vi "Stream Update All Sensors.vi"(8 "error in":errorcluster, 11 "UART port in":T9) -> (0 "error out":errorcluster, 1 "sensors":T1={"Bumps + Wheel Drops"={"Wheeldrop Caster"=FALSE, "Wheeldrop Left"=FALSE, "Wheeldrop Right"=FALSE, "Bump Left"=FALSE, "Bump Right"=FALSE}, "Wall"=FALSE, "Cliff Left"=FALSE, "Cliff Front Left"=FALSE, "Cliff Front Right"=FALSE, "Cliff Right"=FALSE, "Wall Signal"=0, "Cliff Left Signal"=0, "Cliff Front Left Signal"=0, "Cliff Front Right Signal"=0, "Cliff Right Signal"=0, "Buttons"={"Advance"=FALSE, "Play"=FALSE}, "Virtual Wall"=FALSE, "# Stream Packets"=0, "Requested Velocity (mm/s)"=0, "Requested Radius (mm)"=0, "Requested Right Wheel Velocity (mm/s)"=0, "Requested Left Wheel Velocity (mm/s)"=0, "Distance (mm)"=0, "Angle (deg)"=0, "Song Playing"=FALSE, "Song Number"=0, "Charging State"=enum."Not Charging", "Voltage (mV)"=0, "Current (mA)"=0, "Battery Temperature (deg C)"=0, "Battery Charge (mAh)"=0, "Battery Capacity (mAh)"=0, "Charging Sources"={"Internal Charger"=FALSE, "Home Base"=FALSE}, "OI Mode"=enum."Off", "Digital Inputs"={"Digital Input 0"=FALSE, "Digital Input 1"=FALSE, "Digital Input 2"=FALSE, "Digital Input 3"=FALSE, "Device Detect"=FALSE}, "Drivers & Wheel Overcurrent"={"Low-Side Driver 0"=FALSE, "Low-Side Driver 1"=FALSE, "Low-Side Driver 2"=FALSE, "Left Wheel"=FALSE, "Right Wheel"=FALSE}, "Analog Signal"=0, "Infrared"=255} {"Infrared" format="%02x"}, 3 "UART port out":T9, 5 "Accumulated Distance (mm)":i32, 7 "Accumulated Angle (deg)":i32)   [LabVIEW 2013]
doc: "Reads data from the UART serial port and updates sensors when packets are available.\n\nThis VI assumes that the robot is streaming all sensor data (sensor group 6).\n\nThis VI accumulates distance and angle whenever a new packet is received. While this simplifies most code, which depends on how far the robot has moved, the developer must take account for rollover of signed 32-bit integers if the application has a long running time.\n\nNote that accumulated distance and angle tend to be extremeley inaccurate, since the iRobot looses fractional components of each when it sends a sensor update, and updates are sent at a high rate, resulting in significant roundoff error.\n\nThis VI reads from, but does not write to, the serial port."
uses:
  Advanced/UART/iRobot UART Port Type.ctl
  Sensor Group 6.ctl
  Bumps + Wheel Drops.ctl
  Buttons.ctl
  Charging State.ctl
  Charging Sources Available.ctl
  OI Mode.ctl
  Cargo Bay Digital Inputs.ctl
  Low-Side Driver + Wheel Overcurrent.ctl
  Advanced/UART/iRobot UART Simple Packet Configuration.ctl
panel:
  # "Electrical: charging, battery, OI mode"
  # "Sensors: bump, cliff, button, wheel drop, wall, virtual wall"
  # "Motion: distance, angle, requested velocity"
  # "Cargo Bay: I/O, overcurrent, infrared"
  # "Song"
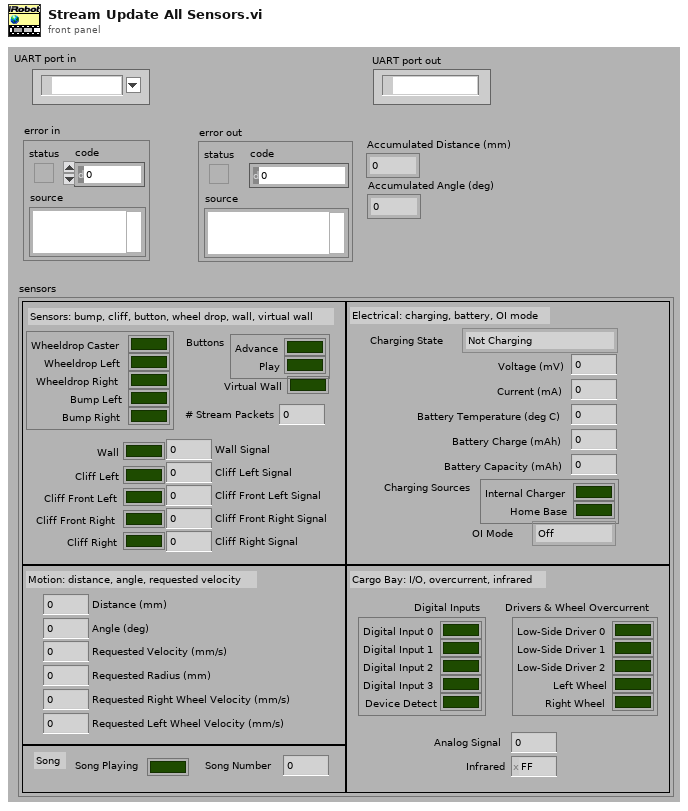
[diagram p1: front panel]
types:
  T1 = typedef "Sensor Group 6.ctl" = cluster{"Bumps + Wheel Drops":T2, "Wall":bool, "Cliff Left":bool, "Cliff Front Left":bool, "Cliff Front Right":bool, "Cliff Right":bool, "Wall Signal":u16, "Cliff Left Signal":u16, "Cliff Front Left Signal":u16, "Cliff Front Right Signal":u16, "Cliff Right Signal":u16, "Buttons":T3, "Virtual Wall":bool, "# Stream Packets":u8, "Requested Velocity (mm/s)":i16, "Requested Radius (mm)":i16, "Requested Right Wheel Velocity (mm/s)":i16, "Requested Left Wheel Velocity (mm/s)":i16, "Distance (mm)":i32, "Angle (deg)":i32, "Song Playing":bool, "Song Number":u8, "Charging State":T4, "Voltage (mV)":u16, "Current (mA)":i16, "Battery Temperature (deg C)":i8, "Battery Charge (mAh)":u16, "Battery Capacity (mAh)":u16, "Charging Sources":T5, "OI Mode":T6, "Digital Inputs":T7, "Drivers & Wheel Overcurrent":T8, "Analog Signal":u16, "Infrared":u8}
  T2 = typedef "Bumps + Wheel Drops.ctl" = cluster{"Wheeldrop Caster":bool, "Wheeldrop Left":bool, "Wheeldrop Right":bool, "Bump Left":bool, "Bump Right":bool}
  T3 = typedef "Buttons.ctl" = cluster{"Advance":bool, "Play":bool}
  T4 = typedef "Charging State.ctl" = enum16{"Not Charging", "Reconditioning Charging", "Full Charging", "Trickle Charging", "Waiting", "Charging Fault Condition"}
  T5 = typedef "Charging Sources Available.ctl" = cluster{"Internal Charger":bool, "Home Base":bool}
  T6 = typedef "OI Mode.ctl" = enum16{"Off", "Passive", "Safe", "Full"}
  T7 = typedef "Cargo Bay Digital Inputs.ctl" = cluster{"Digital Input 0":bool, "Digital Input 1":bool, "Digital Input 2":bool, "Digital Input 3":bool, "Device Detect":bool}
  T8 = typedef "Low-Side Driver + Wheel Overcurrent.ctl" = cluster{"Low-Side Driver 0":bool, "Low-Side Driver 1":bool, "Low-Side Driver 2":bool, "Left Wheel":bool, "Right Wheel":bool}
  T9 = typedef "iRobot UART Port Type.ctl" = refnum<visa-resource-name>
  T10 = typedef "iRobot UART Simple Packet Configuration.ctl" = cluster{"header":u8[], "create checksum?":bool}
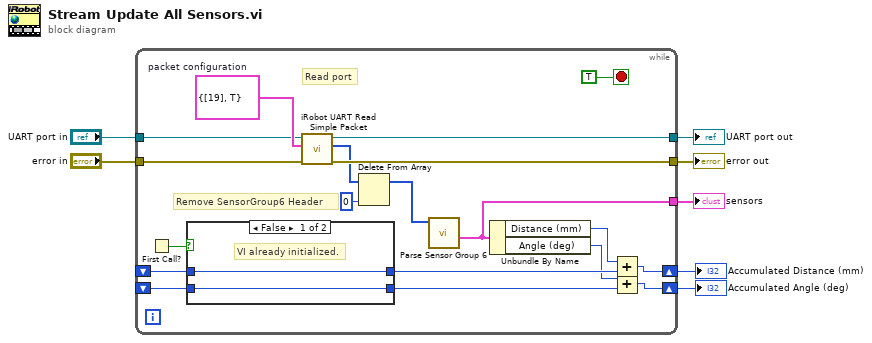
[diagram p0: block diagram]
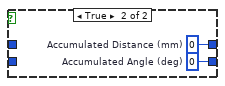
[diagram p2: hidden frame]
diagram:
  n1 = while {
    tunnel: "error in" -> [w13]
    shift-right: [w22] -> w6
    shift-left: _ -> [w20]
    shift-right: [w21] -> w5
    shift-left: _ -> [w19]
    tunnel: [w18] -> w4
    tunnel: [w14] -> w2
    tunnel: "UART port in" -> [w9]
    tunnel: [w8] -> w1
    stop <- TRUE stop-if-true
    w17 = T10 {"header"=[19], "create checksum?"=TRUE}  # packet configuration
    # "Remove SensorGroup6 Header"
    # "Read port"
    n2 = First Call?() -> (First Call?: T/F=w26:bool)
    n3 = case shown="False" w26 {
      tunnel: [w28 w30] -> w24
      tunnel: [w27 w29] -> w23
      tunnel: w20 -> [w28 _]
      tunnel: w19 -> [w27 _]
      frame False {
        # "VI already initialized."
      }
      frame True {
        w29 = 0  # Accumulated Angle (deg)
        w30 = 0  # Accumulated Distance (mm)
      }
    }
    n4 = call "iRobot UART Read Simple Packet.vi"("error in"=w13, "packet configuration"=w17, "UART session"=w9) -> ("error out"=w18:errorcluster, "payload"=w12:u8[], "UART session"=w8:T9)  [unwired: 2 in, 4 out]
    n5 = Delete From Array(array=w12, index=0) -> (array with subset deleted=w10:u8[])  [unwired: 1 in, 1 out]
    n6 = call "Parse Sensor Group 6.vi"("stream in"=w10) -> ("iRobot Sensor Group 6"=w14:T1)  [unwired: 9 in, 1 out]
    n7 = Unbundle By Name(w14) -> ("Distance (mm)"=w16:i32, "Angle (deg)"=w15:i32)
    n8 = Add(x=w16, y=w24) -> (x+y=w22:i32)
    n9 = Add(x=w15, y=w23) -> (x+y=w21:i32)
  }
  "UART port out" <- w1
  "sensors" <- w2
  "error out" <- w4
  "Accumulated Distance (mm)" <- w6
  "Accumulated Angle (deg)" <- w5
